vi "Popup Fixed-Point.vi"(8 "error in (no error)":errorcluster, 9 "Panel":refnum<class "Panel.lvclass">, 10 "String in":string, 11 "Numeric Data Type in":refnum<class "Numeric Data Type.lvclass">) -> (0 "error out":errorcluster, 2 "String out":string, 3 "Numeric Data Type out":refnum<class "Numeric Data Type.lvclass">)   [LabVIEW 2018, in "Numeric Data Type.lvclass"]
uses:
  Numeric Data Type.lvclass
  <vilib>/MGI/Panel Manager/Panel/Panel/Panel.lvclass
  Numeric Data Type.lvclass/Numeric Data Type.ctl
  <vilib>/Utility/miscctls.llb/LVPointTypeDef.ctl
panel:
  in  "Numeric":fxp<+/-,64,32>
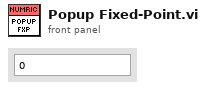
[diagram p1: front panel]
types:
  T1 = typedef "LVPointTypeDef.ctl" = cluster{"Horizontal":i16, "Vertical":i16}
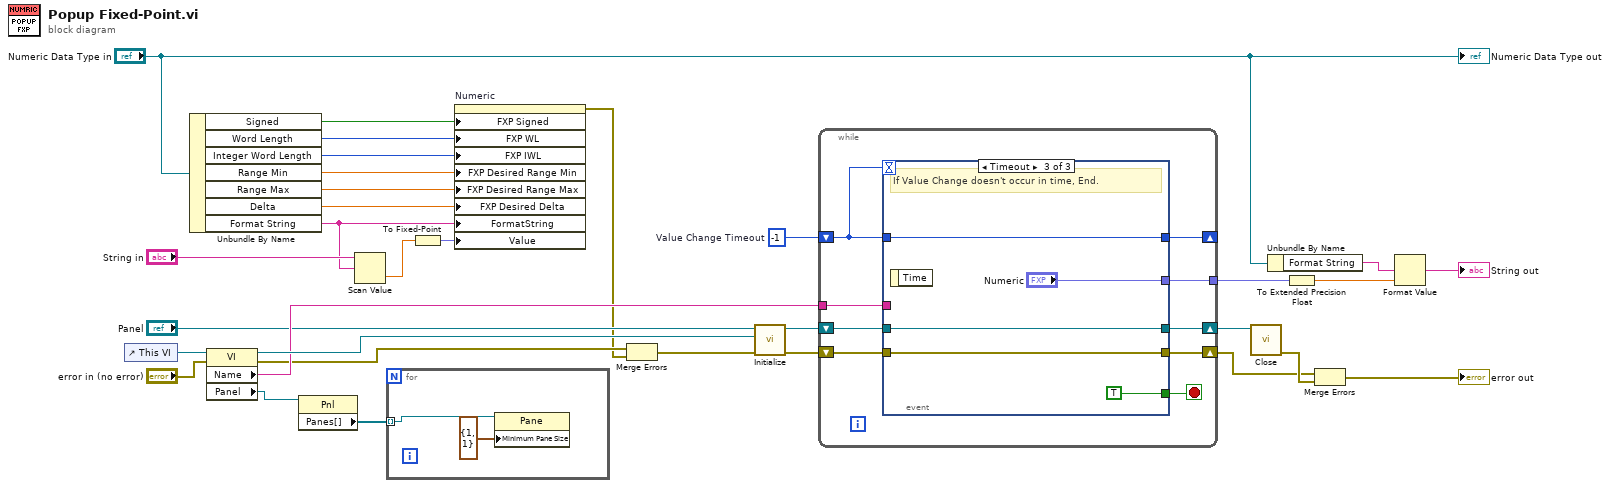
[diagram p0: block diagram]
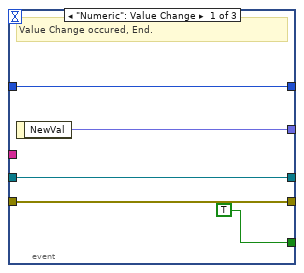
[diagram p2: hidden frame]
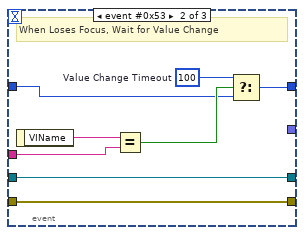
[diagram p3: hidden frame]
diagram:
  w32 = -1  # Value Change Timeout
  n1 = control-ref of="This VI"() -> (w29:refnum<vi>)
  n2 = Unbundle By Name("Numeric Data Type in") -> ("Signed"=w18:bool, "Word Length"=w17:u32, "Integer Word Length"=w16:i32, "Range Min"=w15:dbl, "Range Max"=w14:dbl, "Delta"=w13:dbl, "Format String"=w12:string)
  n3 = property class="VI"(reference=w29, error in="error in (no error)") -> (reference out=w28:refnum<vi>, error out=w20:errorcluster, "Name"=w27:string, "Panel"=w4:refnum<vi>)
  n4 = property class="Pnl"(reference=w4) -> ("Panes[]"=w3:refnum<vi>[])  [unwired: 1 in, 2 out]
  n5 = Scan Value(string="String in", format string=w12) -> (value=w11:dbl)  [unwired: 1 in, 1 out]
  n6 = for {
    tunnel: w3 -> [w34] mode=indexing
    n7 = property class="Pane"(reference=w34, "Minimum Pane Size"=T1 {"Horizontal"=1, "Vertical"=1}) -> ()  [unwired: 1 in, 2 out]
  }
  n8 = To Fixed-Point(number=w11) -> (fixed-point=w1:fxp<+/-,32,16>)  [unwired: 1 in]
  n9 = property on="Numeric" class="DigNum (strict)"("FXP Signed"=w18, "FXP WL"=w17, "FXP IWL"=w16, "FXP Desired Range Min"=w15, "FXP Desired Range Max"=w14, "FXP Desired Delta"=w13, "FormatString"=w12, "Value"=w1) -> (error out=w9:errorcluster)  [unwired: 2 in, 1 out]
  n10 = Merge Errors(w20, w9) -> (w10:errorcluster)
  n11 = call <vilib>:"Initialize.vi"("error in (no error)"=w10, "VI Refnum"=w28, "Panel In"="Panel") -> ("error out"=w30:errorcluster, "Panel Out"=w31:refnum<class "Panel.lvclass">)  [unwired: 6 in, 1 out]
  n12 = while {
    shift-right: [w43] -> w24
    shift-left: w30 -> [w42]
    shift-right: [w40] -> w25
    shift-left: w31 -> [w39]
    tunnel: [w38] -> w8
    tunnel: w27 -> [w37]
    shift-right: [w35] -> _
    shift-left: w32 -> [w36]
    stop <- w41 stop-if-true
    n13 = event shown="[2] Timeout" {
      selector: _ -> [_ _ _]
      dyn-events: _ -> [_ _ _]
      timeout: w36 -> [_ _ _]
      tunnel: [w45 w54 w59] -> w43
      tunnel: w42 -> [w45 w54 w59]
      tunnel: [TRUE _ TRUE] -> w41
      tunnel: [w47 w53 w60] -> w40
      tunnel: w39 -> [w47 w53 w60]
      tunnel: [w46 _ "Numeric"] -> w38
      tunnel: w37 -> [_ w55 _]
      tunnel: w36 -> [w44 w50 w57]
      tunnel: [w44 w49 w57] -> w35
      event "Numeric": Value Change {
        # "Value Change occured, End."
        n14 = event-data() -> ("NewVal"=w46:fxp<+/-,64,32>)  [unwired: 1 in]
      }
      event event #0x53 {
        w51 = 100  # Value Change Timeout
        # "When Loses Focus, Wait for Value Change"
        n15 = event-data() -> ("VIName"=w56:string)  [unwired: 1 in]
        n16 = Equal?(x=w56, y=w55) -> (x = y?=w52:bool)
        n17 = Select(t=w51, s=w52, f=w50) -> (s? t:f=w49:i32)
      }
      event Timeout {
        # "If Value Change doesn't occur in time, End."
        n18 = event-data() -> ()  [unwired: 1 in, 1 out]
      }
    }
  }
  n19 = call-dynamic "Close.vi"("Panel In"=w25) -> ("Error Out"=w26:errorcluster)  [unwired: 10 in]
  n20 = Unbundle By Name("Numeric Data Type in") -> ("Format String"=w6:string)
  n21 = To Extended Precision Float(1:w8) -> (0:w2:ext)
  n22 = Merge Errors(w24, w26) -> (→"error out":errorcluster)
  n23 = Format Value(format string=w6, value (0)=w2) -> (output string=→"String out":string)  [unwired: 1 in]
  "Numeric Data Type out" <- "Numeric Data Type in"
